vi "throw generic error.vi"(8 "error in":errorcluster, 9 "source":string="Throw Generic Error.vi", 10 "append error message":string, 11 "error classification":T1=enum."none") -> (0 "error out":errorcluster)   [LabVIEW 2013, in "TBM module execution interface.lvclass"]
uses:
  TBM module execution interface.lvclass
  error classification.ctl
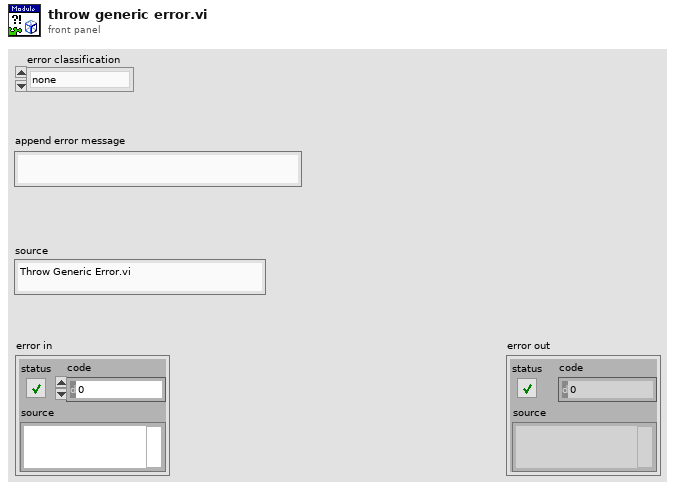
[diagram p1: front panel]
types:
  T1 = typedef "TBM module execution interface.lvclass/error classification.ctl" = enum16{"unknown", "none", "trivial", "recoverable", "critical"}
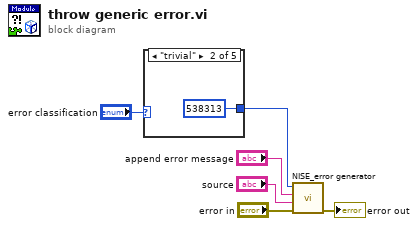
[diagram p0: block diagram]
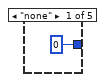
[diagram p2: hidden frame]
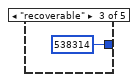
[diagram p3: hidden frame]
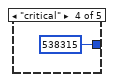
[diagram p4: hidden frame]
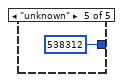
[diagram p5: hidden frame]
diagram:
  n1 = case shown="\"trivial\"" "error classification" {
    tunnel: [0 ("error code (0)") 538313 ("error code (0)") 538314 ("error code (0)") 538315 ("error code (0)") 538312 ("error code (0)")] -> w3
    frame "none" {
    }
    frame "trivial" {
    }
    frame "recoverable" {
    }
    frame "critical" {
    }
    frame "unknown" {
    }
  }
  n2 = call <vilib>:"NISE_error generator.vi"("error in"="error in", "source"="source", "append error message"="append error message", "error code (0)"=w3) -> ("error out"=→"error out":errorcluster)  [unwired: 5 in]
